vi "HIT_Query.vi"(0 "System no.":i32=1 min=1 max=4 step=1, 2 "Table IDs":i32[](array[numeric]), 3 "Without parameter?":bool, 5 "error in":errorcluster, 6 "Xo":i32=1, 7 "N":i32=100, 8 "Nmax":i32=1024) -> (14 "Data":dbl[][](array[numeric]) format="%.2f", 15 "Table names":string[](array[string]), 16 "HIT? string":string, 19 "error out":errorcluster)   [LabVIEW 2020]
doc: "Returns N points of the current lookup table content. N must be less than or equal to Nmax. For large N values, communication timeout must be set long enough, otherwise a comm.error may occur.\n\nC-867:"
panel:
  # "Returns N points of the current lookup table content. N must be less than or equal to Nmax. For large N values, communication \ntimeout must be set long enough, otherwise a comm.error may occur."
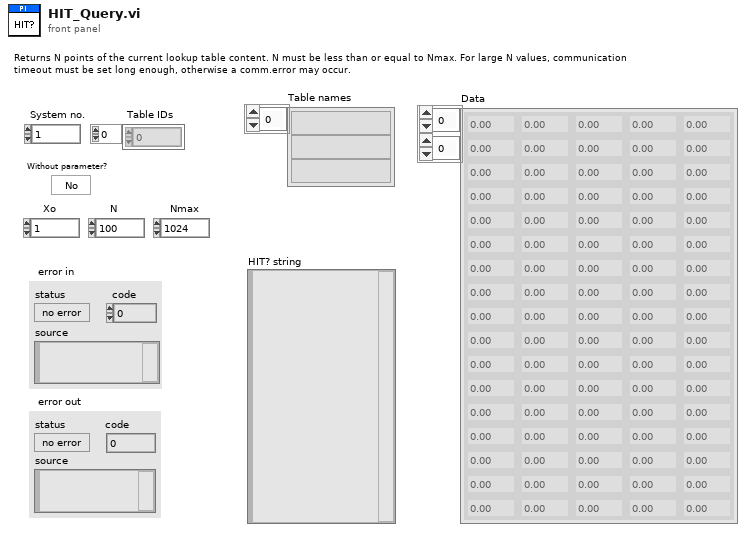
[diagram p1: front panel]
types:
  T1 = cluster{"Read (F)/Write":bool, "Path":path, "Datastream":string, "ArrayName":string}
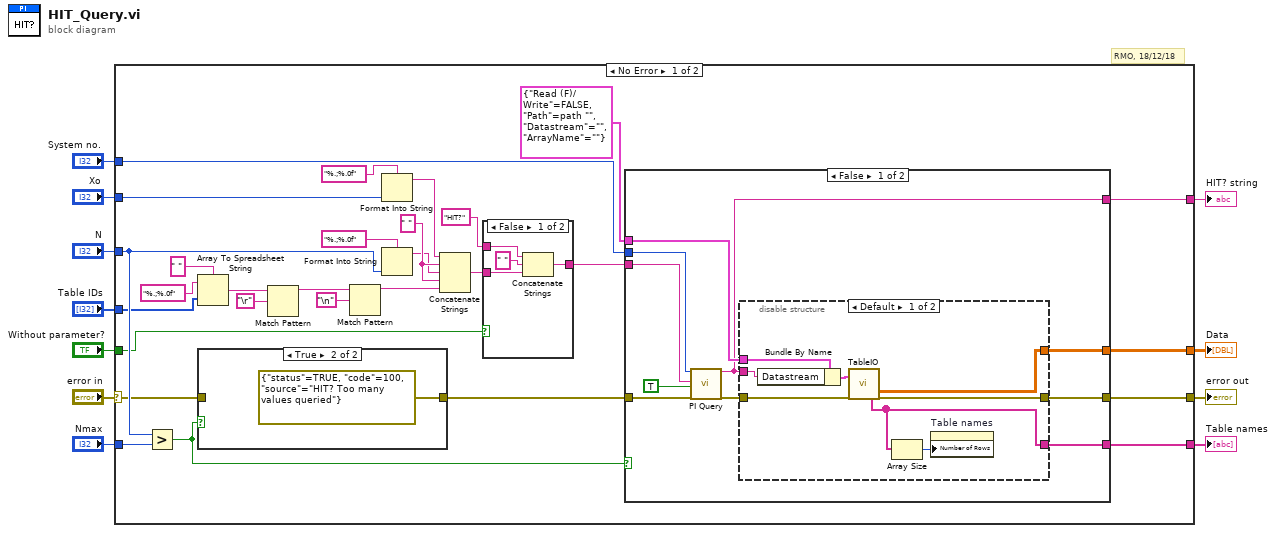
[diagram p0: block diagram]
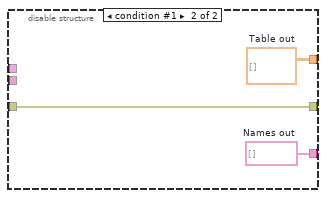
[diagram p3: hidden frame]
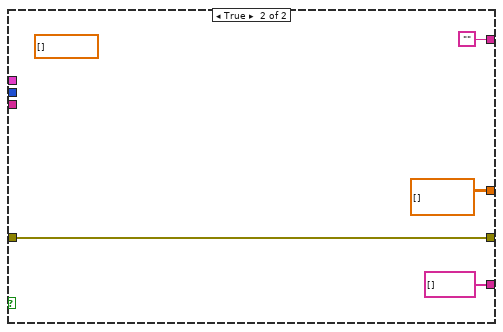
[diagram p4: hidden frame]
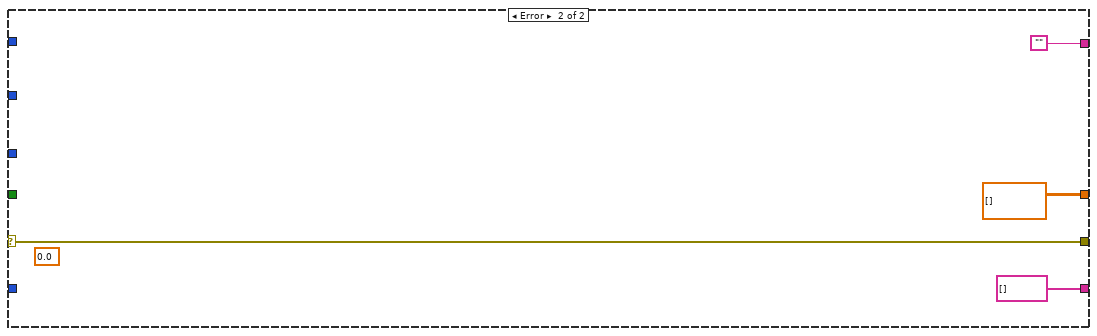
[diagram p6: hidden frame]
diagram:
  # "RMO, 18/12/18"
  n1 = case shown="No Error" "error in" {
    selector: "error in" -> [w12 w73]
    tunnel: "System no." -> [w38 _]
    tunnel: "Table IDs" -> [w20 _]
    tunnel: [w34 w73] -> w10
    tunnel: [w33 dbl[][] [] ("Table out")] -> w6
    tunnel: "N" -> [w28 _]
    tunnel: "Xo" -> [w31 _]
    tunnel: "Nmax" -> [w29 _]
    tunnel: [w26 string[] [] ("Names out")] -> w5
    tunnel: "Without parameter?" -> [w17 _]
    tunnel: [w13 ""] -> w2
    frame No Error {
      w30 = " "
      n2 = Greater?(x=w28, y=w29) -> (0:w35:bool)
      n3 = Array To Spreadsheet String(delimiter (Tab)=" ", array=w20, 3:"%.;%.0f" ("Format String")) -> (spreadsheet string=w15:string)
      n4 = case shown="True" w35 {
        tunnel: [w71 errorcluster {"status"=TRUE, "code"=100, "source"="HIT? Too many values queried"} ("error out")] -> w36
        tunnel: w12 -> [w71 _]
        frame False {
        }
        frame True {
        }
      }
      n5 = Match Pattern(string=w15, regular expression="\r") -> (before substring=w14:string)  [unwired: 4 out]
      n6 = Match Pattern(string=w14, regular expression="\n") -> (before substring=w19:string)  [unwired: 4 out]
      n7 = Format Into String(format string="%.;%.0f" ("Format String"), w31) -> (resulting string=w25:string)  [unwired: 2 in, 1 out]
      n8 = Format Into String(format string="%.;%.0f" ("Format String"), w28) -> (resulting string=w24:string)  [unwired: 2 in, 1 out]
      n9 = Concatenate Strings(w25, w30, w24, w30, w19) -> (w18:string)
      n10 = case shown="False" w17 {
        tunnel: "HIT?" -> [w44 w45]
        tunnel: [w43 w45] -> w39
        tunnel: w18 -> [w42 _]
        frame False {
          n11 = Concatenate Strings(w44, " " ("Substring"), w42) -> (w43:string)
        }
        frame True {
        }
      }
      n12 = case shown="False" w35 {
        tunnel: w39 -> [w54 _]
        tunnel: w38 -> [w53 _]
        tunnel: w36 -> [w50 w70]
        tunnel: [w49 w70] -> w34
        tunnel: [w51 dbl[][] [] ("Table out")] -> w33
        tunnel: T1 {"Read (F)/Write"=FALSE, "Path"=path "", "Datastream"="", "ArrayName"=""} ("IOSource") -> [w52 _]
        tunnel: [w48 string[] [] ("Names out")] -> w26
        tunnel: [w46 ""] -> w13
        frame False {
          n13 = call "PI Query.vi"("System no."=w53, "String to send"=w54, "Attach termination char.?"=TRUE ("Attach Linefeed?"), "error in"=w50) -> ("String read"=w46:string, "error out"=w47:errorcluster)  [unwired: 3 in, 11 out]
          n14 = disable-structure shown="Default" {
            disable-tunnel: w52 -> [w63 _]
            disable-tunnel: [w61 w65] -> w51
            disable-tunnel: w47 -> [w60 w66]
            disable-tunnel: [w59 w66] -> w49
            disable-tunnel: [w57 w64] -> w48
            disable-tunnel: w46 -> [w56 _]
            frame condition #0 (active) {
              n15 = Bundle By Name(cluster=w63, "Datastream"=w56) -> (w62:T1)
              n16 = call "TableIO.vi"("IOSource"=w62, "error in"=w60) -> ("Names out"=w57:string[], "Table out"=w61:dbl[][], "error out"=w59:errorcluster)  [unwired: 4 in, 11 out]
              n17 = Array Size(array=w57) -> (size(s)=w58:i32)
              n18 = property on="Table names" class="Arr (strict)"("Number of Rows"=w58) -> ()  [unwired: 2 in, 2 out]
            }
            frame condition #1 {
              w64 = string[] []  # Names out
              w65 = dbl[][] []  # Table out
            }
          }
        }
        frame True {
          (unwired) dbl[] [] ("Waveform points")
        }
      }
    }
    frame Error {
      (unwired) 0.0 ("Sample Time out")
    }
  }
  "error out" <- w10
  "Data" <- w6
  "Table names" <- w5
  "HIT? string" <- w2
